vi "Boolean Stream Communication.vi"(2 "Mode":T1(ring), 7 "IP 4":i32, 11 "Error In":errorcluster) -> (8 "Calibrated?":bool, 15 "Error Out":errorcluster)   [LabVIEW 2013]
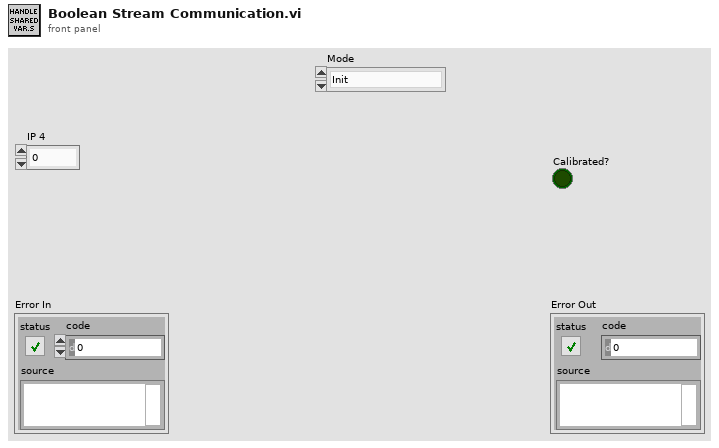
[diagram p1: front panel]
types:
  T1 = enum16{"Init", "Stream Signals", "Stream Calibrated", "Check Stream", "File Trigger"}
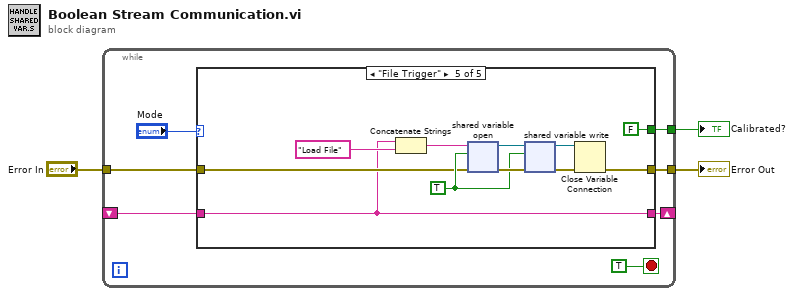
[diagram p0: block diagram]
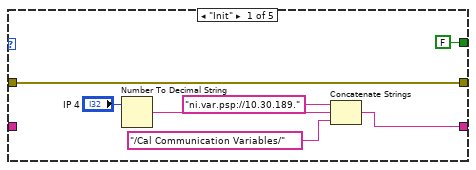
[diagram p2: hidden frame]
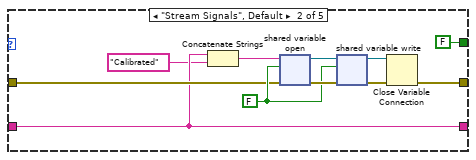
[diagram p3: hidden frame]
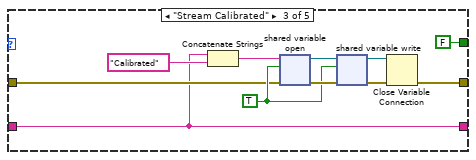
[diagram p4: hidden frame]
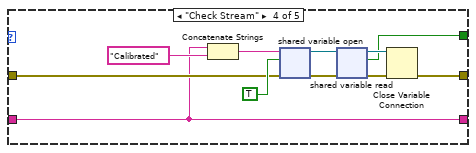
[diagram p5: hidden frame]
diagram:
  n1 = while {
    tunnel: "Error In" -> [w8]
    tunnel: [w7] -> w2
    tunnel: [w6] -> w1
    shift-right: [w5] -> _
    shift-left: _ -> [w4]
    stop <- TRUE stop-if-true
    n2 = case shown="\"File Trigger\"" "Mode" {
      tunnel: w8 -> [w17 w21 w31 w41 w54]
      tunnel: [w17 w24 w36 w50 w61] -> w7
      tunnel: [FALSE FALSE FALSE w44 FALSE] -> w6
      tunnel: [w11 w20 w30 w40 w51] -> w5
      tunnel: w4 -> [_ w20 w30 w40 w51]
      frame "Init" {
        n3 = Number To Decimal String(number="IP 4") -> (decimal integer string=w14:string)  [unwired: 1 in]
        n4 = Concatenate Strings("ni.var.psp://10.30.189.", w14, "/Cal Communication Variables/") -> (w11:string)
      }
      frame "Stream Signals", Default {
        w23 = FALSE
        n5 = Concatenate Strings(w20, "Calibrated") -> (w18:string)
        n6 = shared-variable-open(w18, w21, w23) -> (w28:refnum<k21>, w25:errorcluster)  [unwired: 1 in]
        n7 = shared-variable-write(w28, w25, w23) -> (w27:refnum<k21>, w26:errorcluster)
        n8 = Close Variable Connection(8:w26, 11:w27) -> (0:w24:errorcluster)
      }
      frame "Stream Calibrated" {
        w35 = TRUE
        n9 = Concatenate Strings(w30, "Calibrated") -> (w29:string)
        n10 = shared-variable-open(w29, w31, w35) -> (w33:refnum<k21>, w37:errorcluster)  [unwired: 1 in]
        n11 = shared-variable-write(w33, w37, w35) -> (w39:refnum<k21>, w38:errorcluster)
        n12 = Close Variable Connection(8:w38, 11:w39) -> (0:w36:errorcluster)
      }
      frame "Check Stream" {
        n13 = Concatenate Strings(w40, "Calibrated") -> (w42:string)
        n14 = shared-variable-open(w42, w41, TRUE) -> (w47:refnum<k21>, w48:errorcluster)  [unwired: 1 in]
        n15 = shared-variable-read(w47, w48) -> (w45:refnum<k21>, w46:errorcluster, w44:bool)  [unwired: 1 out]
        n16 = Close Variable Connection(8:w46, 11:w45) -> (0:w50:errorcluster)
      }
      frame "File Trigger" {
        w56 = TRUE
        n17 = Concatenate Strings(w51, "Load File") -> (w52:string)
        n18 = shared-variable-open(w52, w54, w56) -> (w57:refnum<k21>, w60:errorcluster)  [unwired: 1 in]
        n19 = shared-variable-write(w57, w60, w56) -> (w58:refnum<k21>, w59:errorcluster)
        n20 = Close Variable Connection(8:w59, 11:w58) -> (0:w61:errorcluster)
      }
    }
  }
  "Error Out" <- w2
  "Calibrated?" <- w1
